vi "read_params.vi"(8 "error in (no error)":errorcluster, 11 "SpectralClustering in":refnum<class "SpectralClustering.lvclass">) -> (0 "error out":errorcluster, 2 "params":T1={"n_clusters"=8.0, "eigen_solver"="None", "n_components"={"n_components_type"="None", "n_components_int"=8.0}, "random_state"=0.0, "n_init"=10.0, "gamma"=1.0, "affinity"="rbf", "n_neighbors"=10.0, "eigen_tol"=0.0, "assign_labels"="kmeans", "degree"=0.0, "coef0"=1.0, "n_jobs"=1.0, "verbose"=FALSE}, 3 "SpectralClustering out":refnum<class "SpectralClustering.lvclass">)   [LabVIEW 2020, in "SpectralClustering.lvclass"]
uses:
  SpectralClustering.lvclass
  Controls/spectral_clustering_params.ctl
  SpectralClustering.lvclass/SpectralClustering.ctl
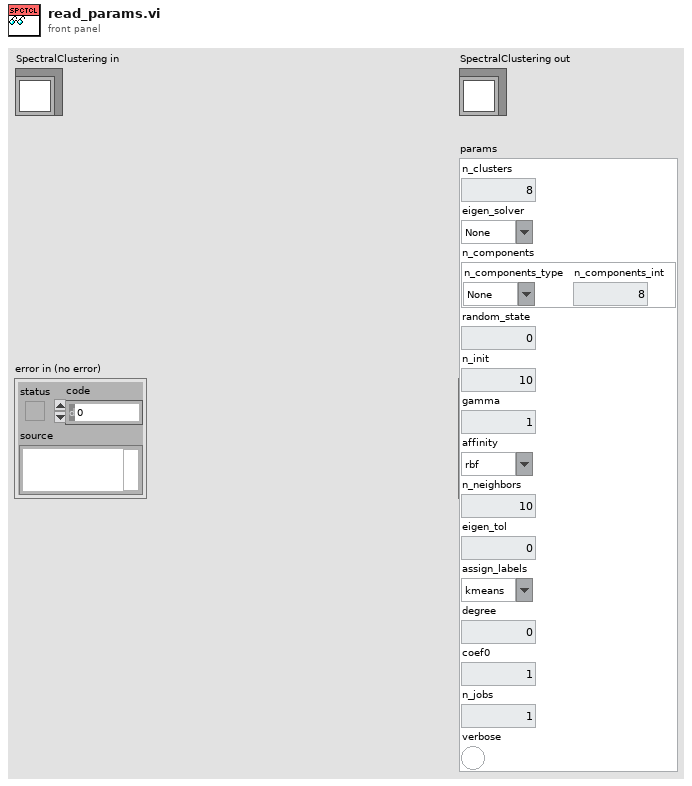
[diagram p1: front panel]
types:
  T1 = typedef "spectral_clustering_params.ctl" = cluster{"n_clusters":dbl, "eigen_solver":string, "n_components":cluster{"n_components_type":string, "n_components_int":dbl}, "random_state":dbl, "n_init":dbl, "gamma":dbl, "affinity":string, "n_neighbors":dbl, "eigen_tol":dbl, "assign_labels":string, "degree":dbl, "coef0":dbl, "n_jobs":dbl, "verbose":bool}
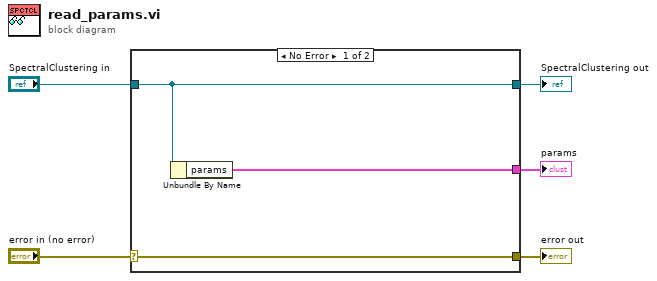
[diagram p0: block diagram]
diagram:
  n1 = case shown="No Error" "error in (no error)" {
    selector: "error in (no error)" -> [w8 w9]
    tunnel: [w8 w9] -> w4
    tunnel: [w7 w10] -> w2
    tunnel: "SpectralClustering in" -> [w7 w10]
    tunnel: [w6 _] -> w1
    frame No Error {
      n2 = Unbundle By Name(w7) -> ("params"=w6:T1)
    }
    frame Error {
    }
  }
  "error out" <- w4
  "SpectralClustering out" <- w2
  "params" <- w1
